vi "getModbusRxDataFIFO.vi"(11 "ILCCommunications in":refnum<class "ILCCommunications.lvclass">) -> (2 "ModbusRxDataFIFO":refnum<class "IReadU16FIFO.lvclass">, 3 "ILCCommunications out":refnum<class "ILCCommunications.lvclass">)   [LabVIEW 2016, in "ILCCommunications.lvclass"]
uses:
  ILCCommunications.lvclass
  Common_RT_FPGA/IReadU16FIFO/IReadU16FIFO.lvclass
  ILCCommunications.lvclass/ILCCommunications.ctl
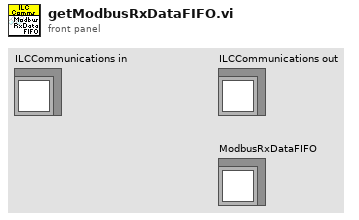
[diagram p1: front panel]
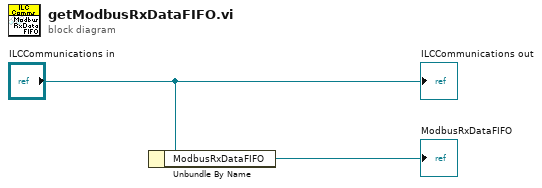
[diagram p0: block diagram]
diagram:
  n1 = Unbundle By Name("ILCCommunications in") -> ("ModbusRxDataFIFO"=→"ModbusRxDataFIFO":refnum<class "IReadU16FIFO.lvclass">)
  "ILCCommunications out" <- "ILCCommunications in"
